vi "Query Trigger Event Overrun.vi"(8 "error in (no error)":errorcluster, 10 "Trigger Event (0: Digital 1)":i32(ring) items=["Digital 1", "Digital 2", "Digital 3", "Digital 4", "Digital 5", "Digital 6", "Timer 1", "Timer 2", "Timer 3", "Timer 4", "Lan 1", "Lan 2", "Lan 3", "Lan 4", "Lan 5", "Lan 6", "Lan 7", "Lan 8", "External In", "Blender 1", "Blender 2"], 11 "VISA resource name":refnum<visa-resource-name>) -> (0 "error out":errorcluster, 2 "Overrun Status (0)":i32, 3 "VISA resource name out":refnum<visa-resource-name>)   [LabVIEW 2020, in "Keithley DMM6500 DAQ6500 Series.lvlib"]
doc: "Queries the trigger event overrun status."
uses:
  <instrlib>/Keithley DMM6500 DAQ6500 Series/Keithley DMM6500 DAQ6500 Series.lvlib
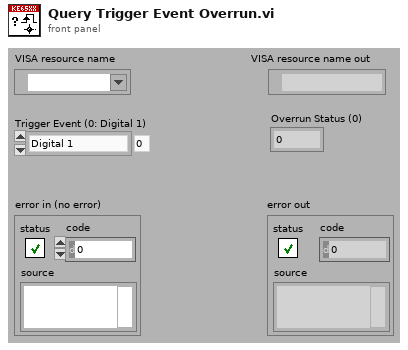
[diagram p1: front panel]
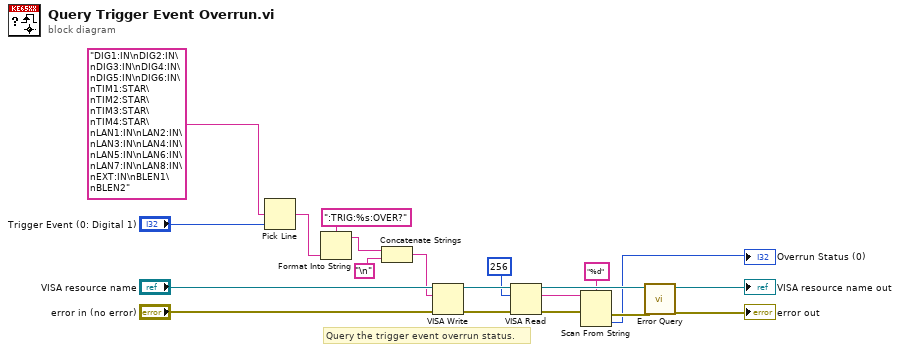
[diagram p0: block diagram]
diagram:
  # "Query the trigger event overrun status."
  n1 = Pick Line(multi-line string="DIG1:IN\nDIG2:IN\nDIG3:IN\nDIG4:IN\nDIG5:IN\nDIG6:IN\nTIM1:STAR\nTIM2:STAR\nTIM3:STAR\nTIM4:STAR\nLAN1:IN\nLAN2:IN\nLAN3:IN\nLAN4:IN\nLAN5:IN\nLAN6:IN\nLAN7:IN\nLAN8:IN\nEXT:IN\nBLEN1\nBLEN2", line index="Trigger Event (0: Digital 1)") -> (output string=w10:string)  [unwired: 1 in]
  n2 = Format Into String(format string=":TRIG:%s:OVER?", w10) -> (resulting string=w13:string)  [unwired: 2 in, 1 out]
  n3 = Concatenate Strings(w13, "\n" ("Line Feed Constant")) -> (w11:string)
  n4 = VISA Write(VISA resource name="VISA resource name", write buffer=w11, error in (no error)="error in (no error)") -> (VISA resource name out=w9:refnum<visa-resource-name>, error out=w8:errorcluster)  [unwired: 1 out]
  n5 = VISA Read(VISA resource name=w9, byte count=u32 256, error in (no error)=w8) -> (VISA resource name out=w4:refnum<visa-resource-name>, read buffer=w2:string, error out=w6:errorcluster)  [unwired: 1 out]
  n6 = Scan From String(format string="%d", input string=w2, error in=w6) -> (error out=w5:errorcluster, output 1=→"Overrun Status (0)":i32)  [unwired: 2 in, 2 out]
  n7 = call <instrlib>:"Error Query.vi"("error in (no error)"=w5, "VISA resource name"=w4) -> ("error out"=→"error out":errorcluster, "VISA resource name out"=→"VISA resource name out":refnum<visa-resource-name>)  [unwired: 6 in, 2 out]
